vi "motor format.vi"(0 "motor array":dbl[](array[numeric])) -> (2 "Center Motor Fill Style":i32, 3 "Center Color":u32(colorbox), 4 "Back Right Motor Fill Style":i32, 6 "Back Right Color":u32(colorbox), 8 "Back Left Motor Fill Style":i32, 10 "Back Left Color":u32(colorbox), 12 "Front Right Color":u32(colorbox), 13 "Front Right Motor Fill Style":i32, 14 "Front Left Color":u32(colorbox), 15 "Front Left Motor Fill Style":i32)   [LabVIEW 2015]
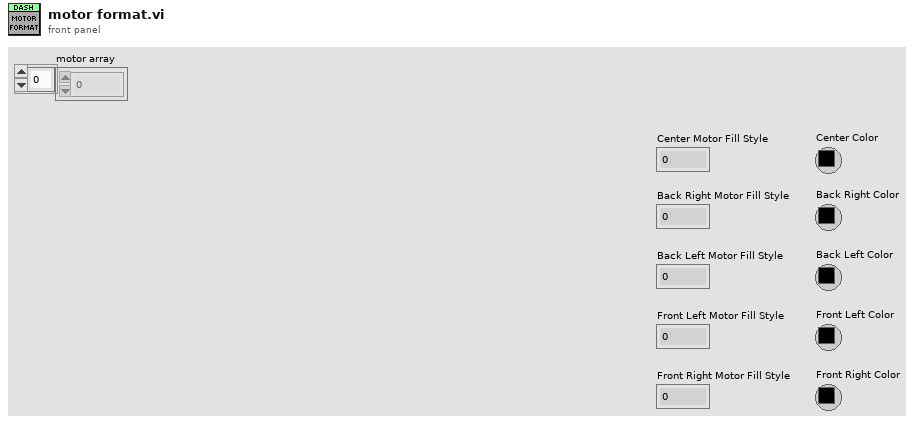
[diagram p1: front panel]
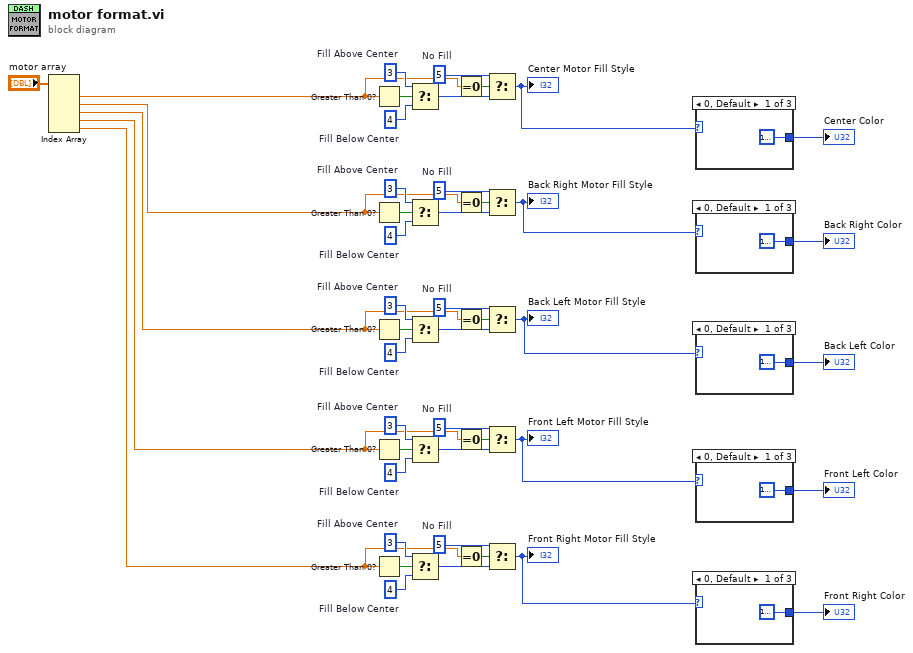
[diagram p0: block diagram]
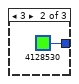
[diagram p2: hidden frame]
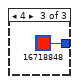
[diagram p3: hidden frame]
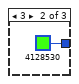
[diagram p4: hidden frame]
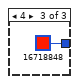
[diagram p5: hidden frame]
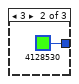
[diagram p6: hidden frame]
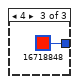
[diagram p7: hidden frame]
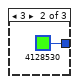
[diagram p8: hidden frame]
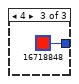
[diagram p9: hidden frame]
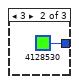
[diagram p10: hidden frame]
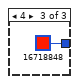
[diagram p11: hidden frame]
diagram:
  w21 = 4  # Fill Below Center
  w20 = 3  # Fill Above Center
  w19 = 5  # No Fill
  w22 = 4  # Fill Below Center
  w23 = 3  # Fill Above Center
  w24 = 5  # No Fill
  w33 = 4  # Fill Below Center
  w32 = 3  # Fill Above Center
  w31 = 5  # No Fill
  w34 = 4  # Fill Below Center
  w35 = 3  # Fill Above Center
  w36 = 5  # No Fill
  w46 = 4  # Fill Below Center
  w45 = 3  # Fill Above Center
  w44 = 5  # No Fill
  n1 = Index Array(array="motor array") -> (element #1=w2:dbl, element #2=w15:dbl, element #3=w14:dbl, element #4=w40:dbl, element #5=w13:dbl)  [unwired: 5 in]
  n2 = Greater Than 0?(x=w2) -> (x > 0?=w27:bool)
  n3 = Greater Than 0?(x=w15) -> (x > 0?=w28:bool)
  n4 = Greater Than 0?(x=w14) -> (x > 0?=w39:bool)
  n5 = Greater Than 0?(x=w40) -> (x > 0?=w41:bool)
  n6 = Greater Than 0?(x=w13) -> (x > 0?=w16:bool)
  n7 = Select(t=w23, s=w27, f=w22) -> (s? t:f=w25:i32)
  n8 = Select(t=w32, s=w28, f=w33) -> (s? t:f=w30:i32)
  n9 = Select(t=w35, s=w39, f=w34) -> (s? t:f=w37:i32)
  n10 = Select(t=w45, s=w41, f=w46) -> (s? t:f=w43:i32)
  n11 = Select(t=w20, s=w16, f=w21) -> (s? t:f=w18:i32)
  n12 = Equal To 0?(x=w2) -> (x = 0?=w26:bool)
  n13 = Equal To 0?(x=w15) -> (x = 0?=w29:bool)
  n14 = Equal To 0?(x=w14) -> (x = 0?=w38:bool)
  n15 = Equal To 0?(x=w40) -> (x = 0?=w42:bool)
  n16 = Equal To 0?(x=w13) -> (x = 0?=w17:bool)
  n17 = Select(t=w24, s=w26, f=w25) -> (s? t:f=w3:i32)
  "Center Motor Fill Style" <- w3
  n18 = Select(t=w31, s=w29, f=w30) -> (s? t:f=w11:i32)
  "Back Right Motor Fill Style" <- w11
  n19 = Select(t=w36, s=w38, f=w37) -> (s? t:f=w10:i32)
  "Back Left Motor Fill Style" <- w10
  n20 = Select(t=w44, s=w42, f=w43) -> (s? t:f=w7:i32)
  "Front Left Motor Fill Style" <- w7
  n21 = Select(t=w19, s=w17, f=w18) -> (s? t:f=w5:i32)
  "Front Right Motor Fill Style" <- w5
  n22 = case shown="0, Default" w3 {
    tunnel: [u32 16777216 ("Center Color") u32 4128530 ("Center Color") u32 16718848 ("Center Color")] -> w12
    frame 0, Default {
    }
    frame 3 {
    }
    frame 4 {
    }
  }
  "Center Color" <- w12
  n23 = case shown="0, Default" w11 {
    tunnel: [u32 16777216 ("Center Color") u32 4128530 ("Center Color") u32 16718848 ("Center Color")] -> w9
    frame 0, Default {
    }
    frame 3 {
    }
    frame 4 {
    }
  }
  "Back Right Color" <- w9
  n24 = case shown="0, Default" w10 {
    tunnel: [u32 16777216 ("Center Color") u32 4128530 ("Center Color") u32 16718848 ("Center Color")] -> w8
    frame 0, Default {
    }
    frame 3 {
    }
    frame 4 {
    }
  }
  "Back Left Color" <- w8
  n25 = case shown="0, Default" w7 {
    tunnel: [u32 16777216 ("Center Color") u32 4128530 ("Center Color") u32 16718848 ("Center Color")] -> w6
    frame 0, Default {
    }
    frame 3 {
    }
    frame 4 {
    }
  }
  "Front Left Color" <- w6
  n26 = case shown="0, Default" w5 {
    tunnel: [u32 16777216 ("Center Color") u32 4128530 ("Center Color") u32 16718848 ("Center Color")] -> w4
    frame 0, Default {
    }
    frame 3 {
    }
    frame 4 {
    }
  }
  "Front Right Color" <- w4
